vi "dfd_FXP Overflow (vector).vi"(4 "quantization settings":T1={"source"=6, "wl"=1, "iwl"=1, "overflow mode"=enum."Saturation", "rounding mode"=enum."Nearest", "signed?"=TRUE} {"source" items=["Coef a/k"=0, "Coef b/v"=7, "Input"=1, "Output"=2, "Multiplicand"=3, "Product"=4, "Sum"=5, "Delay"=6, "Gain"=8]}, 8 "values in":dbl[](array[numeric]) format="%.2f") -> (1 "# underflow":i32, 2 "# overflow":i32, 3 "values out":dbl[](array[numeric]) format="%.2f")   [LabVIEW 2017, in "NI_DigFilter_FXP.lvlib"]
uses:
  <vilib>/addons/Digital Filter Design/NI_DigFilter_FXP.lvlib
  <vilib>/addons/Digital Filter Design/_Objects.llb/dfd_Internal Quantization Settings.ctl
  <vilib>/addons/Digital Filter Design/_Objects.llb/dfd_Internal Quantization Srcs.ctl
  <vilib>/addons/Digital Filter Design/NI_DigFilterLicensed.lvlib
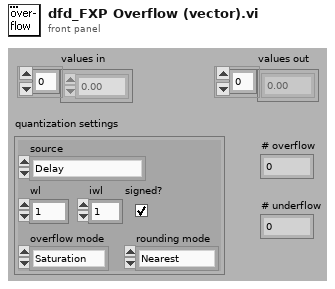
[diagram p1: front panel]
types:
  T1 = typedef "NI_DigFilterLicensed.lvlib/dfd_Internal Quantization Settings.ctl" = cluster{"source":T2, "wl":i16, "iwl":i16, "overflow mode":enum16{"Saturation", "Wrap"}, "rounding mode":enum16{"Nearest", "Truncation"}, "signed?":bool}
  T2 = typedef "NI_DigFilterLicensed.lvlib/dfd_Internal Quantization Srcs.ctl" = u16
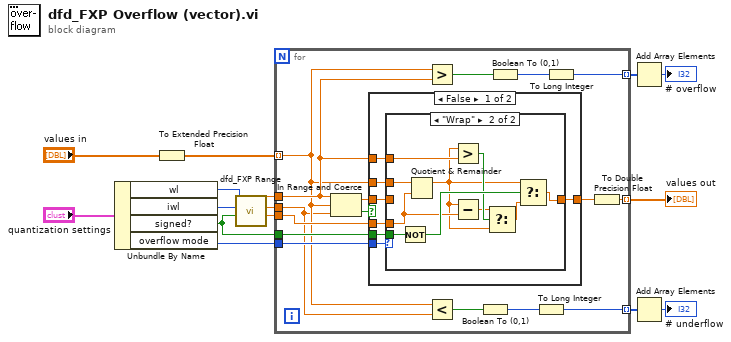
[diagram p0: block diagram]
diagram:
  n1 = Unbundle By Name("quantization settings") -> ("wl"=w2:i16, "iwl"=w1:i16, "signed?"=w13:bool, "overflow mode"=w15:enum16{"Saturation", "Wrap"})
  n2 = To Extended Precision Float(1:"values in") -> (0:w9:ext[])
  n3 = call <vilib>:"dfd_FXP Range.vi"("signed?"=w13, "iwl"=w1, "wl"=w2) -> ("full range"=w14:ext, "low"=w8:ext, "high"=w11:ext)  [unwired: 6 out]
  n4 = for {
    tunnel: w15 -> [w29]
    tunnel: w14 -> [w28]
    tunnel: w13 -> [w27]
    tunnel: w11 -> [w26]
    tunnel: [w23] -> w10 mode=indexing
    tunnel: w9 -> [w22] mode=indexing
    tunnel: w8 -> [w21]
    tunnel: [w20] -> w7 mode=indexing
    tunnel: [w16] -> w5 mode=indexing
    n5 = In Range and Coerce(upper limit=w26, x=w22, lower limit=w21) -> (coerced(x)=w30:ext, In Range?=w31:bool)
    n6 = case shown="False" w31 {
      tunnel: [w36 w50] -> w17
      tunnel: w30 -> [w37 w50]
      tunnel: w29 -> [w38 _]
      tunnel: w28 -> [w35 _]
      tunnel: w22 -> [w34 _]
      tunnel: w27 -> [w33 _]
      tunnel: w26 -> [w32 _]
      frame False {
        n7 = case shown="\"Wrap\"" w38 {
          tunnel: [w39 w48] -> w36
          tunnel: w37 -> [w39 _]
          tunnel: w35 -> [_ w42]
          tunnel: w34 -> [_ w49]
          tunnel: w33 -> [_ w47]
          tunnel: w32 -> [_ w45]
          frame "Saturation", Default {
          }
          frame "Wrap" {
            n8 = Not(x=w47) -> (.not. x?=w46:bool)
            n9 = Quotient & Remainder(x=w49, y=w42) -> (x-y*floor(x/y)=w41:ext)  [unwired: 1 out]
            n10 = Greater?(x=w41, y=w45) -> (0:w44:bool)
            n11 = Subtract(x=w41, y=w42) -> (x-y=w43:ext)
            n12 = Select(t=w43, s=w44, f=w41) -> (s? t:f=w40:ext)
            n13 = Select(t=w41, s=w46, f=w40) -> (s? t:f=w48:ext)
          }
        }
      }
      frame True {
      }
    }
    n14 = Greater?(x=w22, y=w26) -> (0:w24:bool)
    n15 = Less?(x=w22, y=w21) -> (x < y?=w18:bool)
    n16 = Boolean To (0,1)(Boolean=w18) -> (0, 1=w19:i16)
    n17 = Boolean To (0,1)(Boolean=w24) -> (0, 1=w25:i16)
    n18 = To Long Integer(number=w19) -> (32bit integer=w20:i32)
    n19 = To Long Integer(number=w25) -> (32bit integer=w23:i32)
    n20 = To Double Precision Float(number=w17) -> (double precision float=w16:dbl)
  }
  "values out" <- w5
  n21 = Add Array Elements(numeric array=w10) -> (sum=→"# overflow":i32)
  n22 = Add Array Elements(numeric array=w7) -> (sum=→"# underflow":i32)
